vi "ModbusCRC32Calculator.vi"(11 "ModbusCRC32Settings":T1={"DataFIFO"="MockGyroCRCDataFIFO", "CalculateFIFO"="MockGyroCRCCalculateFIFO", "OutputFIFO"="MockGyroCRCFIFO"}) -> ()   [LabVIEW 2016]
uses:
  ModbusCRC32Settings.ctl
  <vilib>/rvi/Emulation/niFpgaGetClockAttributes.vi
  <vilib>/rvi/Emulation/niFpgaSctlEmulationGetInTimedLoop.vi
  <vilib>/rvi/Emulation/niFpgaEmulationReportErrorSimple.vi
  <vilib>/rvi/DataTransferAndStorage/Container/Common/niFpgaContainerExecOnDevCompGetState.vi
  <vilib>/rvi/Emulation/niFpgaEmulationIsFPGAContextNoSignature.vi
  <vilib>/rvi/errors/niFpgaSetErrorForExecOnDevCompSimple.vi
  <vilib>/rvi/eio/common/nirviEmuReportErrorAndStop.vi
  <vilib>/rvi/DataTransferAndStorage/Container/Common/niFpgaContainerGetUniqueNameForEmu.vi
  <vilib>/rvi/FIFO/Fifo_Resource/nirvififoEmulationSetSize.vi
  <vilib>/rvi/FIFO/Fifo_Resource/nirviFifoEmulationQueueMgr.vi
  <instcachedir>/0/nirviFifoEmulationQueueMgr_E5CAEC123FF24DC58D834DCA3CDAA9B5.lvgen/nirviFifoEmulationQueueMgr_E5CAEC123FF24DC58D834DCA3CDAA9B5_000.vi
  <vilib>/rvi/FIFO/Fifo_Resource/nirvififoEmulationDetermineInputValidOut.vi
  <vilib>/rvi/FIFO/Fifo_Resource/nirvififoEmulationCreateLock.vi
  <vilib>/rvi/Emulation/niFpgaProcessEmulError.vi
  <vilib>/rvi/FIFO/Fifo_Resource/nirvififoEmulationObtainLock.vi
  <vilib>/rvi/FIFO/Fifo_Resource/nirvififoEmulationReleaseLock.vi
  <vilib>/rvi/occurrence/nirviWaitOnOccurrenceBase.vi
  <vilib>/rvi/errors/nirviReportUnexpectedCaseInternalError.vi
  <vilib>/rvi/errors/nirviReportUnexpectedCaseInternalError (U32).vi
  <vilib>/Utility/error.llb/Clear Errors.vi
  <vilib>/rvi/interface/RandomDataEmulation/niFpgaRandomDataHandleErrors.vi
  <instcachedir>/0/nirviFifoEmulationQueueMgr_E5CAEC123FF24DC58D834DCA3CDAA9B5.lvgen/nirviFifoEmulationQueueMgr_E5CAEC123FF24DC58D834DCA3CDAA9B5_001.vi
  <vilib>/rvi/Emulation/niFpgaCriticalErrorInLSC.vi
  <vilib>/rvi/DataTransferAndStorage/Container/XNode/niFpgaContainer.xnode
  <vilib>/rvi/FIFO/Fifo_Resource/niFpgaFifoEmulationRefIn.vi
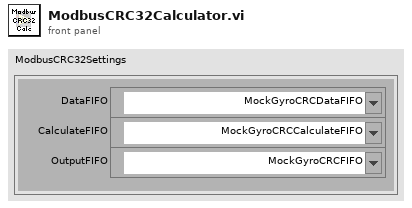
[diagram p1: front panel]
types:
  T1 = typedef "ModbusCRC32Settings.ctl" = cluster{"DataFIFO":refnum<k21>, "CalculateFIFO":refnum<k21>, "OutputFIFO":refnum<k21>}
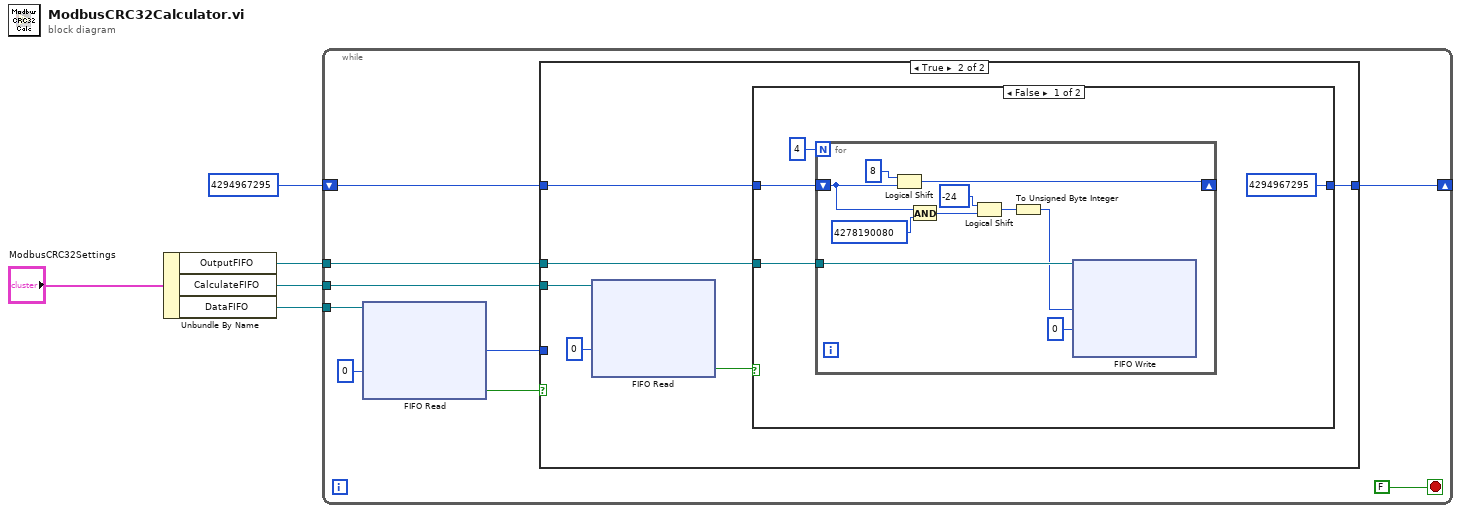
[diagram p0: block diagram]
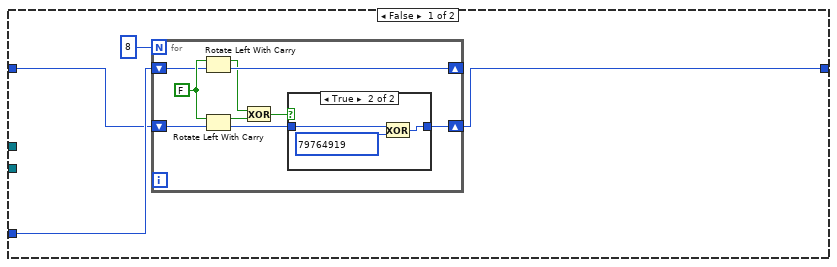
[diagram p2: hidden frame]
diagram:
  n1 = Unbundle By Name("ModbusCRC32Settings") -> ("OutputFIFO"=w5:refnum<k21>, "CalculateFIFO"=w4:refnum<k21>, "DataFIFO"=w3:refnum<k21>)
  n2 = while {
    tunnel: w5 -> [w6]
    tunnel: w4 -> [w7]
    tunnel: w3 -> [w13]
    shift-right: [w8] -> _
    shift-left: u32 4294967295 ("Initial CRC") -> [w10]
    stop <- FALSE stop-if-true
    n3 = xnode ("FIFO Read")("Timeout"=0, "FIFO In"=w13) -> ("Element"=w9:u8, "Timed Out?"=w11:bool)  [unwired: 1 out]
    n4 = case shown="True" w11 {
      tunnel: w10 -> [w16 w35]
      tunnel: w9 -> [w17 _]
      tunnel: [w15 w34] -> w8
      tunnel: w7 -> [_ w37]
      tunnel: w6 -> [_ w33]
      frame False {
        n5 = for {
          N: 8 -> [_]
          shift-right: [w22] -> w15
          shift-left: w16 -> [w20]
          shift-right: [w25] -> _
          shift-left: w17 -> [w26]
          w27 = FALSE ("carry")
          n6 = Rotate Left With Carry(2:w26, 3:w27) -> (0:w25:u8, 1:w24:bool)
          n7 = Rotate Left With Carry(2:w20, 3:w27) -> (0:w19:u32, 1:w21:bool)
          n8 = Exclusive Or(1:w21, 2:w24) -> (0:w23:bool)
          n9 = case shown="True" w23 {
            tunnel: w19 -> [w28 w31]
            tunnel: [w28 w30] -> w22
            frame False {
            }
            frame True {
              n10 = Exclusive Or(1:u32 79764919, 2:w31) -> (0:w30:u32)
            }
          }
        }
      }
      frame True {
        n11 = xnode ("FIFO Read")("Timeout"=0, "FIFO In"=w37) -> ("Timed Out?"=w32:bool)  [unwired: 2 out]
        n12 = case shown="False" w32 {
          tunnel: w35 -> [w40 w52]
          tunnel: [u32 4294967295 ("Initial CRC") w52] -> w34
          tunnel: w33 -> [w38 _]
          frame False {
            n13 = for {
              N: 4 -> [_]
              shift-right: [w50] -> _
              shift-left: w40 -> [w48]
              tunnel: w38 -> [w47]
              n14 = Logical Shift(y=i16 8, x=w48) -> (x << y=w50:u32)
              n15 = And(x=w48, y=u32 4278190080) -> (x .and. y?=w45:u32)
              n16 = Logical Shift(y=i16 -24, x=w45) -> (x << y=w44:u32)
              n17 = To Unsigned Byte Integer(number=w44) -> (unsigned 8bit integer=w42:u8)
              n18 = xnode ("FIFO Write")("Element"=w42, "Timeout"=0, "FIFO In"=w47) -> ()  [unwired: 2 out]
            }
          }
          frame True {
          }
        }
      }
    }
  }
